vi "Vector2DScale.vi"(9 "Scale Factor":dbl, 10 "Vector":T1) -> (2 "Scaled Vector":T1)   [LabVIEW 2018]
uses:
  Vector2D.ctl
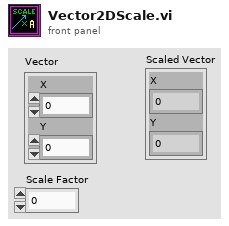
[diagram p1: front panel]
types:
  T1 = typedef "Vector2D.ctl" = cluster{"X":dbl, "Y":dbl}
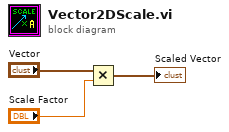
[diagram p0: block diagram]
diagram:
  n1 = Multiply(x="Vector", y="Scale Factor") -> (x*y=→"Scaled Vector":T1)
